vi "Read ADC.vi"(8 "error in (no error)":errorcluster, 9 "Canal":u8, 10 "VISA resource name":refnum<visa-resource-name>, 11 "Simulated in":refnum<class "Simulated.lvclass">) -> (0 "error out":errorcluster, 1 "Response":i32, 2 "VISA resource name 2":refnum<visa-resource-name>, 3 "Simulated out":refnum<class "Simulated.lvclass">, 4 "String":string)   [LabVIEW 2020, in "Simulated.lvclass"]
uses:
  Simulated.lvclass
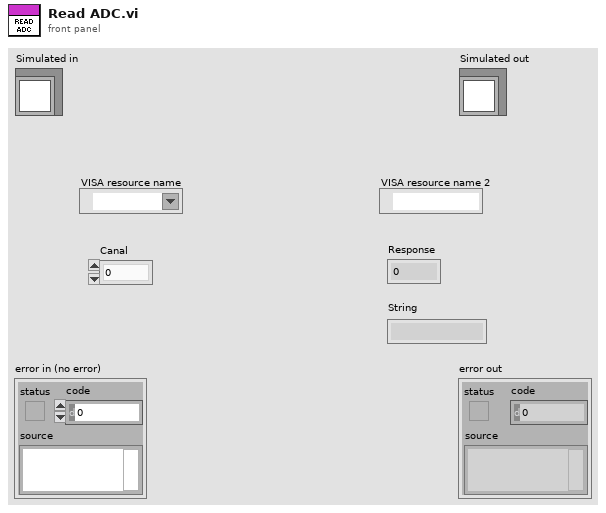
[diagram p1: front panel]
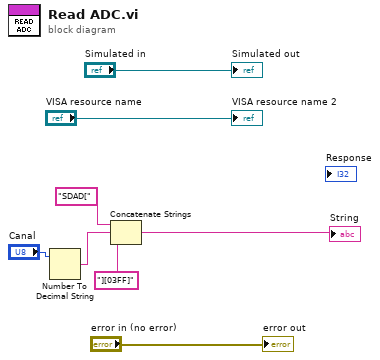
[diagram p0: block diagram]
diagram:
  n1 = Number To Decimal String(number="Canal") -> (decimal integer string=w3:string)  [unwired: 1 in]
  n2 = Concatenate Strings("SDAD[" ("string"), w3, "][03FF]" ("string")) -> (→"String":string)
  "error out" <- "error in (no error)"
  "Simulated out" <- "Simulated in"
  "VISA resource name 2" <- "VISA resource name"
